vi "Launcher.vi"() -> ()   [LabVIEW 2019]
panel:
  out "Engines Firing":bool
  out "Engine Shutoff Timer":dbl
  out "Countdown":dbl
  in  "Abort":bool
  in  "Launch":bool
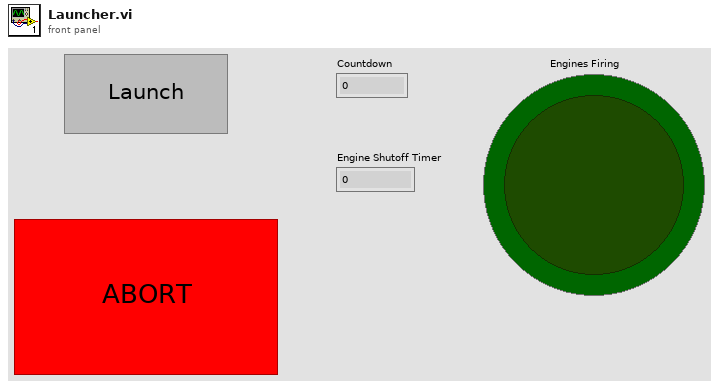
[diagram p1: front panel]
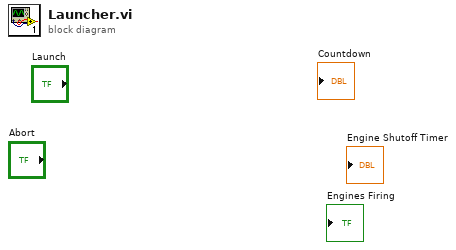
[diagram p0: block diagram]
diagram:
